vi "Identify Projections.vi"(10 "Projection Info":T1[](array[typedef]), 11 "Class Ref Map":variant) -> (2 "Projection Ref Map":variant, 3 "Class Ref Map Dup":variant)   [LabVIEW 2013]
uses:
  Data Structures/JSON/Projection Info.ctl
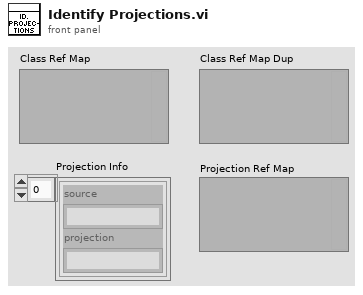
[diagram p1: front panel]
types:
  T1 = typedef "Projection Info.ctl" = cluster{"source":string, "projection":string}
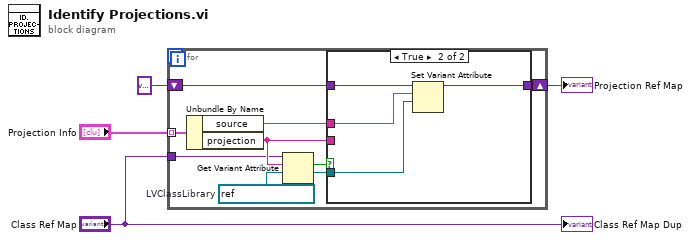
[diagram p0: block diagram]
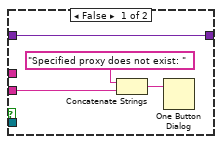
[diagram p2: hidden frame]
diagram:
  n1 = for {
    tunnel: "Projection Info" -> [w13] mode=indexing
    shift-right: [w9] -> w1
    shift-left: variant ("Variant") -> [w8]
    tunnel: "Class Ref Map" -> [w10]
    w6 = refnum<vi> refnum  # LVClassLibrary
    n2 = Unbundle By Name(w13) -> ("source"=w7:string, "projection"=w11:string)
    n3 = Get Variant Attribute(Variant=w10, name=w11, default value (empty Variant)=w6) -> (found=w12:bool, value=w5:refnum<vi>)  [unwired: 1 in, 2 out]
    n4 = case shown="True" w12 {
      tunnel: w11 -> [w16 _]
      tunnel: [w14 w20] -> w9
      tunnel: w8 -> [w14 w21]
      tunnel: w7 -> [_ w19]
      tunnel: w5 -> [_ w18]
      frame False {
        n5 = Concatenate Strings("Specified proxy does not exist: ", w16) -> (w15:string)
        n6 = One Button Dialog(message=w15) -> ()  [unwired: 1 in, 1 out]
      }
      frame True {
        n7 = Set Variant Attribute(Variant=w21, name=w19, value=w18) -> (Variant out=w20:variant)  [unwired: 1 in, 2 out]
      }
    }
  }
  "Projection Ref Map" <- w1
  "Class Ref Map Dup" <- "Class Ref Map"
